vi "Render Node.vi"(6 "Loader":refnum<class "Loader.lvclass">, 8 "Error In":errorcluster, 10 "Node":refnum<class "Node.lvclass">, 11 "Context In":refnum<class "Context.lvclass">) -> (0 "Error Out":errorcluster, 2 "Output":string, 3 "Context Out":refnum<class "Context.lvclass">)   [LabVIEW 2018, in "Toolkit.lvlib"]
uses:
  Toolkit.lvlib
  Context/Context/Context.lvclass
  Nodes/Node/Node.lvclass
  Loaders/Loader/Loader.lvclass
  Nodes/Comment/Comment.lvclass
  Nodes/Delimiter/Delimiter.lvclass
  Nodes/Partial/Partial.lvclass
  Nodes/Section/Section.lvclass
  Nodes/Text/Text.lvclass
  Nodes/Variable/Variable.lvclass
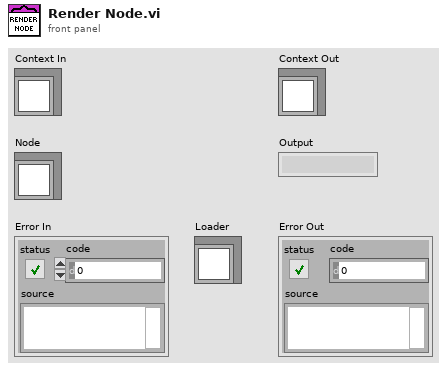
[diagram p1: front panel]
types:
  T1 = typedef "Toolkit.lvlib/Nodes.lvlib/Types.ctl" = enum16{"Comment", "Delimiter", "Partial", "Root", "Section", "Text", "Unknown", "Variable"}
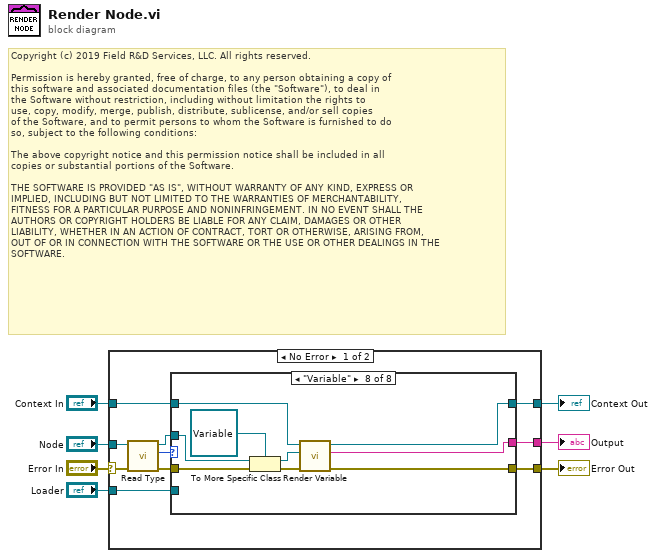
[diagram p0: block diagram]
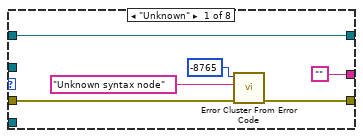
[diagram p2: hidden frame]
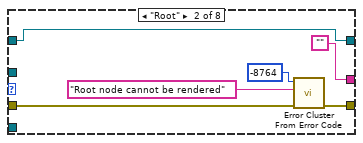
[diagram p3: hidden frame]
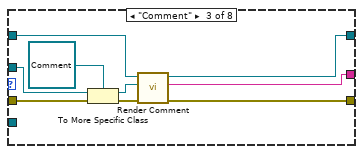
[diagram p4: hidden frame]
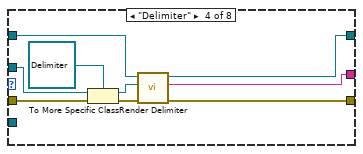
[diagram p5: hidden frame]
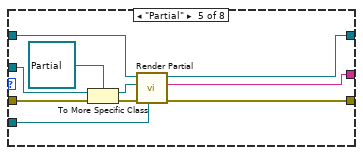
[diagram p6: hidden frame]
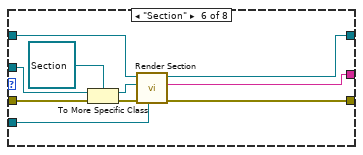
[diagram p7: hidden frame]
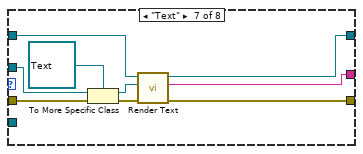
[diagram p8: hidden frame]
diagram:
  # "Copyright (c) 2019 Field R&D Services, LLC. All rights reserved.\n\nPermission is hereby granted, free of charge, to any person obtaining a copy of\nthis software and associated documentation files (the \"Software\"), to deal in\nthe Software without restriction, including without limitation the rights to\nuse, copy, modify, merge, publish, distribute, sublicense, and/or sell copies\nof the Software, and to permit persons to whom the Software is furnished to do\nso, subject to the following conditions:\n\nThe above copyright notice and this permission notice shall be included in all\ncopies or substantial portions of the Software.\n\nTHE SOFTWARE IS PROVIDED \"AS IS\", WITHOUT WARRANTY OF ANY KIND, EXPRESS OR\nIMPLIED, INCLUDING BUT NOT LIMITED TO THE WARRANTIES OF MERCHANTABILITY,\nFITNESS FOR A PARTICULAR PURPOSE AND NONINFRINGEMENT. IN NO EVENT SHALL THE\nAUTHORS OR COPYRIGHT HOLDERS BE LIABLE FOR ANY CLAIM, DAMAGES OR OTHER\nLIABILITY, WHETHER IN AN ACTION OF CONTRACT, TORT OR OTHERWISE, ARISING FROM,\nOUT OF OR IN CONNECTION WITH THE SOFTWARE OR THE USE OR OTHER DEALINGS IN THE\nSOFTWARE."
  n1 = case shown="No Error" "Error In" {
    selector: "Error In" -> [w10 w86]
    tunnel: [w17 w87] -> w7
    tunnel: "Context In" -> [w16 w87]
    tunnel: [w15 _] -> w5
    tunnel: "Node" -> [w14 _]
    tunnel: [w13 w86] -> w3
    tunnel: "Loader" -> [w8 _]
    frame No Error {
      n2 = call-dynamic "Read Type.vi"("Error In"=w10, "Node In"=w14) -> ("Error Out"=w9:errorcluster, "Type"=w11:T1, "Node Out"=w12:refnum<class "Node.lvclass">)  [unwired: 7 in]
      n3 = case shown="\"Variable\"" w11 {
        tunnel: w9 -> [w21 w25 w38 w47 w57 w67 w75 w83]
        tunnel: [w20 w24 w37 w46 w50 w66 w68 w77] -> w13
        tunnel: w12 -> [_ _ w35 w44 w56 w64 w76 w84]
        tunnel: ["" "" w32 w42 w51 w62 w71 w78] -> w15
        tunnel: w16 -> [w23 w29 w31 w41 w53 w61 w70 w80]
        tunnel: [w23 w29 w30 w40 w52 w60 w69 w79] -> w17
        tunnel: w8 -> [_ _ _ _ w48 w58 _ _]
        frame "Unknown" {
          n4 = call <vilib>:"Error Cluster From Error Code.vi"("error in (no error)"=w21, "error message (\"\")"="Unknown syntax node" ("error message (\"\")"), "error code (0)"=-8765) -> ("error out"=w20:errorcluster)  [unwired: 6 in]
        }
        frame "Root" {
          n5 = call <vilib>:"Error Cluster From Error Code.vi"("error in (no error)"=w25, "error message (\"\")"="Root node cannot be rendered" ("error message (\"\")"), "error code (0)"=-8764) -> ("error out"=w24:errorcluster)  [unwired: 6 in]
        }
        frame "Comment" {
          n6 = To More Specific Class(target class=refnum<class "Comment.lvclass"> refnum ("Toolkit.lvlib:Nodes.lvlib:Comment.lvclass"), reference=w35, error in=w38) -> (specific class reference=w33:refnum<class "Comment.lvclass">, error out=w36:errorcluster)
          n7 = call "Render Comment.vi"("Error In"=w36, "Comment"=w33, "Context In"=w31) -> ("Error Out"=w37:errorcluster, "Output"=w32:string, "Context Out"=w30:refnum<class "Context.lvclass">)  [unwired: 6 in]
        }
        frame "Delimiter" {
          n8 = To More Specific Class(target class=refnum<class "Delimiter.lvclass"> refnum ("Toolkit.lvlib:Nodes.lvlib:Delimiter.lvclass"), reference=w44, error in=w47) -> (specific class reference=w43:refnum<class "Delimiter.lvclass">, error out=w45:errorcluster)
          n9 = call "Render Delimiter.vi"("Error In"=w45, "Delimiter"=w43, "Context In"=w41) -> ("Error Out"=w46:errorcluster, "Output"=w42:string, "Context Out"=w40:refnum<class "Context.lvclass">)  [unwired: 6 in]
        }
        frame "Partial" {
          n10 = To More Specific Class(target class=refnum<class "Partial.lvclass"> refnum ("Toolkit.lvlib:Nodes.lvlib:Partial.lvclass"), reference=w56, error in=w57) -> (specific class reference=w49:refnum<class "Partial.lvclass">, error out=w54:errorcluster)
          n11 = call "Render Partial.vi"("Loader"=w48, "Error In"=w54, "Partial"=w49, "Context In"=w53) -> ("Error Out"=w50:errorcluster, "Output"=w51:string, "Context Out"=w52:refnum<class "Context.lvclass">)  [unwired: 5 in]
        }
        frame "Section" {
          n12 = To More Specific Class(target class=refnum<class "Section.lvclass"> refnum ("Toolkit.lvlib:Nodes.lvlib:Section.lvclass"), reference=w64, error in=w67) -> (specific class reference=w63:refnum<class "Section.lvclass">, error out=w65:errorcluster)
          n13 = call "Render Section.vi"("Loader"=w58, "Error In"=w65, "Section"=w63, "Context In"=w61) -> ("Error Out"=w66:errorcluster, "Output"=w62:string, "Context Out"=w60:refnum<class "Context.lvclass">)  [unwired: 5 in]
        }
        frame "Text" {
          n14 = To More Specific Class(target class=refnum<class "Text.lvclass"> refnum ("Toolkit.lvlib:Nodes.lvlib:Text.lvclass"), reference=w76, error in=w75) -> (specific class reference=w72:refnum<class "Text.lvclass">, error out=w73:errorcluster)
          n15 = call "Render Text.vi"("Error In"=w73, "Text"=w72, "Context In"=w70) -> ("Error Out"=w68:errorcluster, "Content"=w71:string, "Context Out"=w69:refnum<class "Context.lvclass">)  [unwired: 6 in]
        }
        frame "Variable" {
          n16 = To More Specific Class(target class=refnum<class "Variable.lvclass"> refnum ("Toolkit.lvlib:Nodes.lvlib:Tag.lvclass"), reference=w84, error in=w83) -> (specific class reference=w81:refnum<class "Variable.lvclass">, error out=w82:errorcluster)
          n17 = call "Render Variable.vi"("Error In"=w82, "Tag"=w81, "Context In"=w80) -> ("Error Out"=w77:errorcluster, "Output"=w78:string, "Context Out"=w79:refnum<class "Context.lvclass">)  [unwired: 6 in]
        }
      }
    }
    frame Error {
    }
  }
  "Context Out" <- w7
  "Output" <- w5
  "Error Out" <- w3
